vi "Initialise.vi"(7 "error in (no error)":errorcluster, 10 "Pre-populated Variant":variant) -> (0 "error out":errorcluster, 3 "ByRef Variant Repsitory out":refnum<data-value>)   [LabVIEW 2015, in "ByRef Variant Repository.lvlib"]
uses:
  ByRef Variant Repository.lvlib
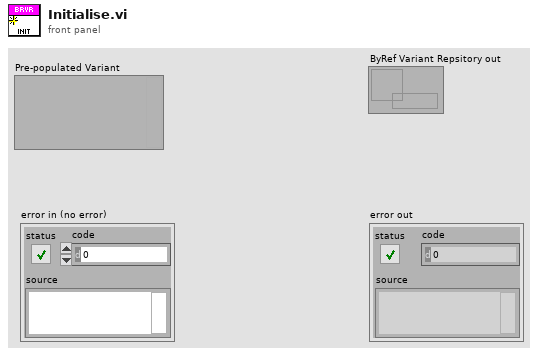
[diagram p1: front panel]
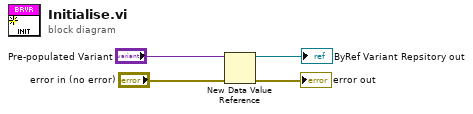
[diagram p0: block diagram]
diagram:
  n1 = New Data Value Reference(data value="Pre-populated Variant", error in="error in (no error)") -> (data value reference=→"ByRef Variant Repsitory out":refnum<data-value>, error out=→"error out":errorcluster)
